vi "Acquire Image from Camera and Save to Image or Video LV2012 NIVerified.vi"() -> ()   [LabVIEW 2012]
doc: "Demonstrates how to acquire images and save them to series of images or a video\n\nLabVIEW can save a video to a AVI container with different kind of codecs. IMAQ AVI2 Get Codec Names returns all available codecs on the system.\nAlternatively the videos single images can be saved to a series of enumerated images with BMP, JPG or PNG format."
uses:
  <vilib>/userdefined/High Color/IMAQdx.ctl
  <vilib>/vision/driver/IMAQdx.llb/IMAQdx Acquisition Mode.ctl
  <vilib>/vision/driver/IMAQdx.llb/IMAQdx Buffer Number Mode.ctl
  <vilib>/vision/driver/NI_Vision_Acquisition_Software.lvlib
panel:
  in  "File Format":enum16{"AVI", "BMP", "JPG", "PNG"}(ring)
  in  "File Name":string
  in  "File Path":path
  in  "stop":bool
  in  "Camera Name":T1
  out "Image":T2(plugin-control)
  out "Buffer Number":u32
  out "Event Overrun":bool
  # "Overview: Demonstrates how to acquire images and save them to series of images or a video\nRequirements: LabVIEW 2012 Base Development System (or compatible)\n                             Vision Development Module 2012 (or compatible)\n                             NI-IMAQdx 4.0 (or compatible)\nInstructions: \n1. Select the file format to save the images to \n2. Select the path where the file(s) are saved to\n3. Select the file name\n4. Select the camera name\n5. Run the VI"
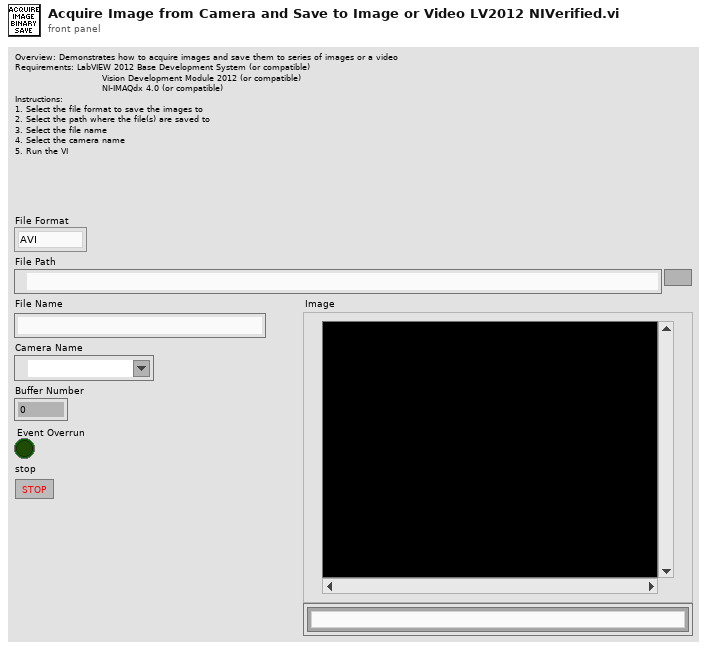
[diagram p1: front panel]
types:
  T1 = typedef "IMAQdx.ctl" = refnum<k21>
  T2 = typedef "IMAQ Image.ctl" = refnum<image>
  T3 = typedef "NI_Vision_Acquisition_Software.lvlib/IMAQdx Acquisition Mode.ctl" = enum32{"One Shot", "Continuous"}
  T4 = typedef "IMAQ AVI2 Refnum.ctl" = refnum<k20>
  T5 = typedef "NI_Vision_Acquisition_Software.lvlib/IMAQdx Buffer Number Mode.ctl" = enum32{"Next", "Last", "Buffer Number"}
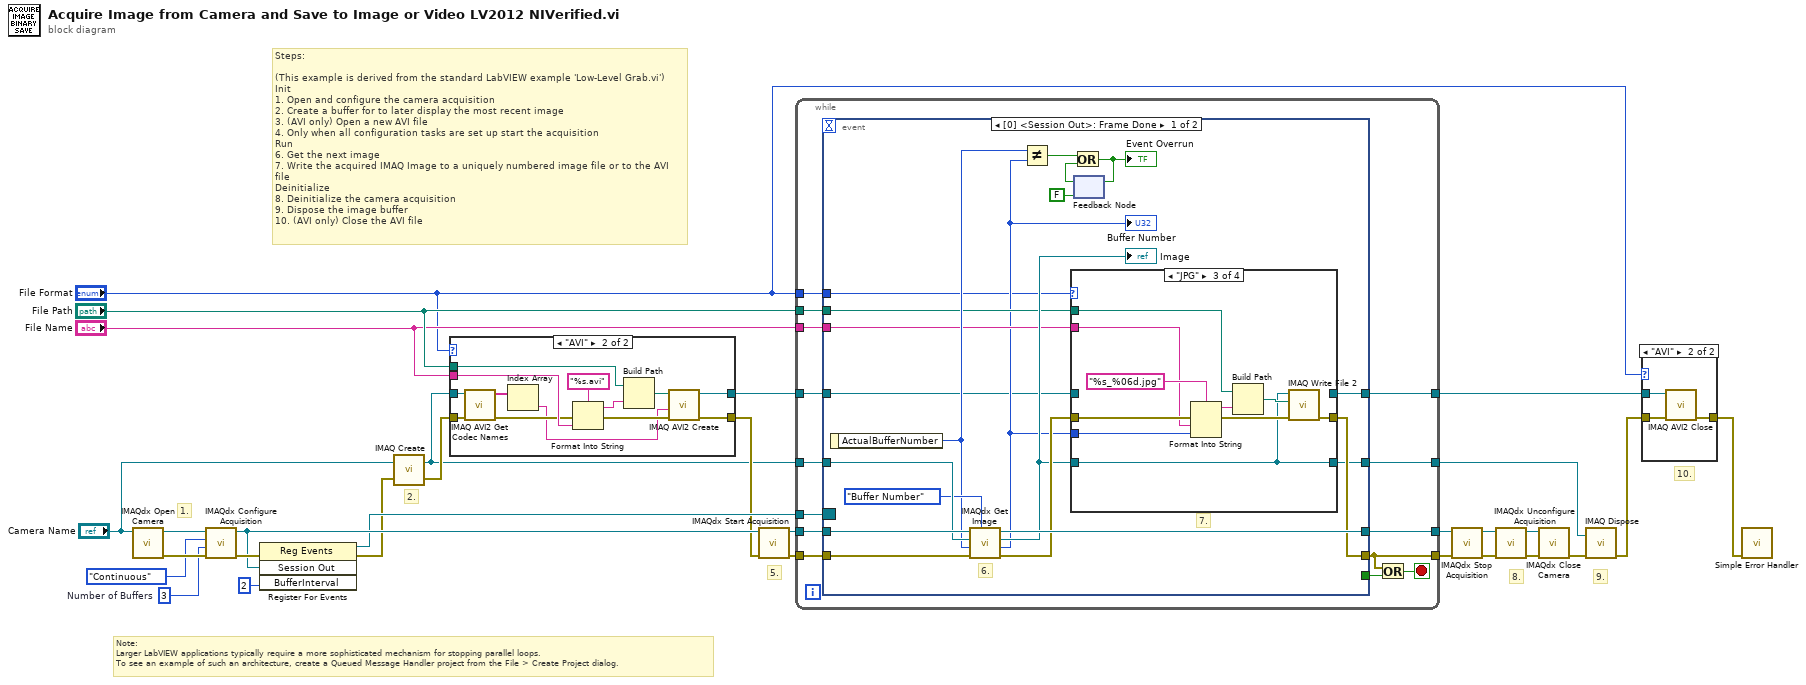
[diagram p0: block diagram]
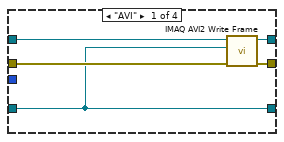
[diagram p4: hidden frame]
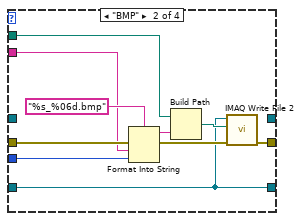
[diagram p5: hidden frame]
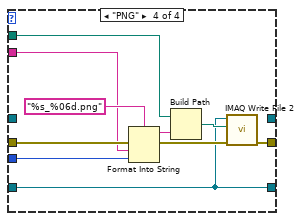
[diagram p6: hidden frame]
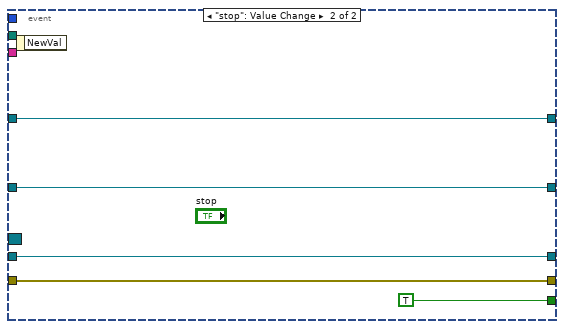
[diagram p7: hidden frame]
diagram:
  w25 = u32 3  # Number of Buffers
  # "Note:\nLarger LabVIEW applications typically require a more sophisticated mechanism for stopping parallel loops.\nTo see an example of such an architecture, create a Queued Message Handler project from the File > Create Project dialog."
  # "9."
  # "10."
  # "8."
  # "5."
  # "2."
  # "1."
  # "Steps:\n\n(This example is derived from the standard LabVIEW example 'Low-Level Grab.vi')\nInit\n1. Open and configure the camera acquisition\n2. Create a buffer for to later display the most recent image\n3. (AVI only) Open a new AVI file\n4. Only when all configuration tasks are set up start the acquisition\nRun\n6. Get the next image\n7. Write the acquired IMAQ Image to a uniquely numbered image file or to the AVI file\nDeinitialize\n8. Deinitialize the camera acquisition\n9. Dispose the image buffer\n10. (AVI only) Close the AVI file"
  n1 = call <vilib>:"IMAQdx Open Camera.vi"("Session In"="Camera Name") -> ("error out"=w27:errorcluster, "Session Out"=w29:T1)  [unwired: 2 in, 7 out]
  n2 = call <vilib>:"IMAQdx Configure Acquisition.vi"("error in"=w27, "Number of Buffers"=w25, "Continuous?"=IMAQdx_Acquisition_Mode."Continuous", "Session In"=w29) -> ("error out"=w18:errorcluster, "Session Out"=w17:T1)  [unwired: 6 out]
  n3 = register-events(error in=w18, w17, u32 2 ("BufferInterval")) -> (reference out=w15:refnum<event-registration>, error out=w14:errorcluster)  [unwired: 1 in]
  n4 = call "IMAQ Create"("Image Name"="Camera Name", "error in (no error)"=w14) -> ("New Image"=w3:T2, "error out"=w4:errorcluster)  [unwired: 2 in, 1 out]
  n5 = case shown="\"AVI\"" "File Format" {
    tunnel: w4 -> [w31 w33]
    tunnel: [w31 w43] -> w12
    tunnel: "File Path" -> [_ w41]
    tunnel: [_ w40] -> w10
    tunnel: "File Name" -> [_ w39]
    tunnel: w3 -> [_ w32]
    frame Default {
    }
    frame "AVI" {
      n6 = call "IMAQ AVI2 Get Codec Names"("error in (no error)"=w33, "Image"=w32) -> ("error out"=w36:errorcluster, "Codec Names"=w35:string[])  [unwired: 8 in]
      n7 = Index Array(array=w35) -> (element=w34:string)  [unwired: 1 in]
      n8 = Format Into String(format string="%s.avi", error in=w36, w39) -> (resulting string=w42:string, error out=w37:errorcluster)  [unwired: 1 in]
      n9 = Build Path(base path=w41, name or relative path=w42) -> (appended path=w38:path)
      n10 = call "IMAQ AVI2 Create"("error in (no error)"=w37, "Codec"=w34, "AVI Path"=w38) -> ("error out"=w43:errorcluster, "AVI Refnum"=w40:T4)  [unwired: 7 in]
    }
  }
  n11 = call <vilib>:"IMAQdx Start Acquisition.vi"("error in"=w12, "Session In"=w17) -> ("error out"=w13:errorcluster, "Session Out"=w28:T1)  [unwired: 8 out]
  n12 = while {
    tunnel: [w54] -> w23
    tunnel: w13 -> [w56]
    tunnel: w28 -> [w57]
    tunnel: [w51] -> w24
    tunnel: w3 -> [w55]
    tunnel: w15 -> [w53]
    tunnel: "File Path" -> [w50]
    tunnel: "File Name" -> [w49]
    tunnel: "File Format" -> [w48]
    tunnel: w10 -> [w47]
    tunnel: [w46] -> w9
    tunnel: [w45] -> w2
    stop <- w58 stop-if-true
    n13 = event shown="[0] <Session Out>: Frame Done" {
      selector: w53 -> [_ _]
      dyn-events: _ -> [_ _]
      timeout: _ -> [_ _]
      tunnel: w57 -> [w78 w116]
      tunnel: w56 -> [w77 w117]
      tunnel: w55 -> [w76 w113]
      tunnel: [w75 w116] -> w54
      tunnel: [w67 w117] -> w51
      tunnel: [_ TRUE] -> w52
      tunnel: w50 -> [w65 _]
      tunnel: w49 -> [w64 _]
      tunnel: w48 -> [w62 _]
      tunnel: w47 -> [w61 w114]
      tunnel: [w60 w114] -> w46
      tunnel: [w59 w113] -> w45
      event event #0x0 {
        # "7."
        # "6."
        n14 = event-data() -> ("ActualBufferNumber"=w73:u32)  [unwired: 1 out]
        n15 = call <vilib>:"IMAQdx Get Image.vi"("Buffer Number Mode (Next)"=IMAQdx_Buffer_Number_Mode."Buffer Number", "error in"=w77, "Buffer Number In"=w73, "Image In"=w76, "Session In"=w78) -> ("error out"=w68:errorcluster, "Buffer Number Out"=w63:u32, "Image Out"=w66:T2, "Session Out"=w75:T1)  [unwired: 3 out]
        "Image" <- w66
        "Buffer Number" <- w63
        n16 = Not Equal?(x=w73, y=w63) -> (x != y?=w72:bool)
        n17 = case shown="\"JPG\"" w62 {
          tunnel: w68 -> [w81 w92 w102 w112]
          tunnel: [w81 w91 w101 w111] -> w67
          tunnel: w66 -> [w79 w83 w93 w103]
          tunnel: w65 -> [_ w87 w97 w107]
          tunnel: w64 -> [_ w85 w95 w105]
          tunnel: w63 -> [_ w84 w94 w104]
          tunnel: w61 -> [w82 _ _ _]
          tunnel: [w80 _ _ _] -> w60
          tunnel: [w79 w83 w93 w103] -> w59
          frame "AVI" {
            n18 = call "IMAQ AVI2 Write Frame"("error in (no error)"=w81, "Image"=w79, "AVI Refnum"=w82) -> ("AVI Refnum (duplicate)"=w80:T4)  [unwired: 6 in, 2 out]
          }
          frame "BMP" {
            n19 = Format Into String(format string="%s_%06d.bmp", error in=w92, w85, w84) -> (resulting string=w88:string, error out=w90:errorcluster)  [unwired: 1 in]
            n20 = Build Path(base path=w87, name or relative path=w88) -> (appended path=w89:path)
            n21 = call-poly "IMAQ Write File 2"("error in (no error)"=w90, "File Path"=w89, "Image"=w83) -> ("error out"=w91:errorcluster)  [unwired: 7 in, 1 out]
          }
          frame "JPG" {
            n22 = Format Into String(format string="%s_%06d.jpg", error in=w102, w95, w94) -> (resulting string=w98:string, error out=w100:errorcluster)  [unwired: 1 in]
            n23 = Build Path(base path=w97, name or relative path=w98) -> (appended path=w99:path)
            n24 = call-poly "IMAQ Write File 2"("error in (no error)"=w100, "File Path"=w99, "Image"=w93) -> ("error out"=w101:errorcluster)  [unwired: 7 in, 1 out]
          }
          frame "PNG" {
            n25 = Format Into String(format string="%s_%06d.png", error in=w112, w105, w104) -> (resulting string=w108:string, error out=w110:errorcluster)  [unwired: 1 in]
            n26 = Build Path(base path=w107, name or relative path=w108) -> (appended path=w109:path)
            n27 = call-poly "IMAQ Write File 2"("error in (no error)"=w110, "File Path"=w109, "Image"=w103) -> ("error out"=w111:errorcluster)  [unwired: 7 in, 1 out]
          }
        }
        n28 = feedback #1(FALSE) -> (w71:bool)
        n29 = Or(x=w72, y=w71) -> (x .or. y?=w70:bool)
        "Event Overrun" <- w70
        n30 = feedback-in #1(w70) -> ()
      }
      event "stop": Value Change {
        n31 = event-data() -> ()  [unwired: 2 out]
      }
    }
    n32 = Or(x=w51, y=w52) -> (x .or. y?=w58:bool)
  }
  n33 = call <vilib>:"IMAQdx Stop Acquisition.vi"("error in"=w24, "Session In"=w23) -> ("error out"=w19:errorcluster, "Session Out"=w20:T1)  [unwired: 8 out]
  n34 = call <vilib>:"IMAQdx Unconfigure Acquisition.vi"("error in"=w19, "Session In"=w20) -> ("error out"=w22:errorcluster, "Session Out"=w21:T1)  [unwired: 8 out]
  n35 = call <vilib>:"IMAQdx Close Camera.vi"("error in"=w22, "Session In"=w21) -> ("error out"=w6:errorcluster)  [unwired: 9 out]
  n36 = call "IMAQ Dispose"("Image"=w2, "error in (no error)"=w6) -> ("error out"=w5:errorcluster)  [unwired: 4 in]
  n37 = case shown="\"AVI\"" "File Format" {
    tunnel: w9 -> [_ w121]
    tunnel: w5 -> [w118 w120]
    tunnel: [w118 w119] -> w8
    frame Default {
    }
    frame "AVI" {
      n38 = call "IMAQ AVI2 Close"("error in (no error)"=w120, "AVI Refnum"=w121) -> ("error out"=w119:errorcluster)  [unwired: 9 in]
    }
  }
  n39 = call <vilib>:"Simple Error Handler.vi"("error in (no error)"=w8) -> ()  [unwired: 4 in, 5 out]
